vi "main.vi"() -> ()   [LabVIEW 2013]
panel:
  in  "?":enum32{"Movement", "Temprature", "Acceleration"}(tab)
  in  "?":dbl
  in  "?":dbl
  in  "?":dbl
  in  "?":dbl
  in  "?":dbl
  in  "?":dbl
  in  "?":dbl
  in  "?":dbl
  in  "?":dbl
  in  "?":dbl
  in  "?":dbl
  in  "?":dbl
  in  "?":dbl
  in  "?":dbl
  in  "?":dbl
  in  "?":dbl
  out "Ch8 2":dbl
  out "Ch7 2":dbl
  out "Ch6 2":dbl
  out "Ch5 2":dbl
  out "Ch4 2":dbl
  out "Ch3 2":dbl
  out "Ch2 2":dbl
  out "Ch1 2":dbl
  out "?":bool
  in  "?":bool
  in  "?":dbl
  in  "?":dbl
  in  "?":dbl
  in  "?":dbl
  in  "?":dbl
  in  "?":dbl
  in  "?":dbl
  in  "?":dbl
  in  "?":dbl
  in  "?":dbl
  in  "?":dbl
  in  "?":dbl
  in  "?":dbl
  in  "?":dbl
  in  "?":dbl
  in  "?":dbl
  out "Ch8":dbl
  out "Ch7":dbl
  out "Ch6":dbl
  out "Ch5":dbl
  out "Ch4":dbl
  out "Ch3":dbl
  out "Ch2":dbl
  out "Ch1":dbl
  out "Strain Graph":waveform(dbl)(graph)
  out "Live Preview":u8[][](graph)
  in  "Blank Button 6":bool
  in  "?":T1(tab)
  in  "Blank Button 2":bool
  in  "Blank Button":bool
  out "Current Position X & Y (units)":dbl[](array[numeric]) format="%_10e"
  out "Postion After Movment  X & Y (units)":dbl[](array[numeric]) format="%_10e"
  in  "Target Displacement X & Y (units)":dbl[](array[numeric]) format="%_6f"
  in  "?":bool
  in  "?":bool
  out "Best Focus":cluster{"X":dbl, "Y":dbl}[](graph)
  in  "Blank Button 5":bool
  in  "Blank Button 4":bool
  in  "Blank Button 3":bool
  in  "?":bool
  in  "?":bool
  out "Postion After Movment Z":dbl format="%_10e"
  in  "Target Displacement Z":dbl format="%_6f"
  out "Current Position Z":dbl format="%_10e"
  out "String":string
  in  "OK Button 17":bool
  in  "OK Button 16":bool
  in  "Sensors 2":T2(radio)
  in  "OK Button 15":bool
  out "?":dbl[](array[numeric]) format="%.6f"
  in  "OK Button 14":bool
  in  "OK Button 13":bool
  in  "OK Button 12":bool
  in  "OK Button 11":bool
  in  "OK Button 10":bool
  in  "OK Button 9":bool
  in  "OK Button 8":bool
  in  "OK Button 7":bool
  in  "OK Button 6":bool
  in  "OK Button 5":bool
  in  "OK Button 4":bool
  in  "OK Button 3":bool
  in  "OK Button 2":bool
  in  "OK Button":bool
  in  "target w 2":dbl=0.2 format="%.6f"
  in  "target v 2":dbl=0.2 format="%.6f"
  in  "target u 2":dbl=0.2 format="%.6f"
  in  "target z 2":dbl=0.2 format="%.6f"
  in  "target y 2":dbl=0.2 format="%.6f"
  in  "target x 2":dbl=0.2 format="%.6f"
  out "current position 3":dbl[](array[numeric]) format="%.6f"
  out "current position 2":dbl[](array[numeric]) format="%.6f"
  out "current position":dbl[](array[numeric]) format="%.6f"
  out "?":dbl[](array[numeric]) format="%.6f"
  in  "target w":dbl=0.2 format="%.6f"
  in  "target v":dbl=0.2 format="%.6f"
  in  "target u":dbl=0.2 format="%.6f"
  in  "target z":dbl=0.2 format="%.6f"
  in  "target y":dbl=0.2 format="%.6f"
  in  "target x":dbl=0.2 format="%.6f"
  in  "Range w":dbl=0.2 format="%.6f"
  in  "Range v":dbl=0.2 format="%.6f"
  in  "Range u":dbl=0.2 format="%.6f"
  in  "Range z":dbl=0.2 format="%.6f"
  in  "Range y":dbl=0.2 format="%.6f"
  in  "Range x":dbl=0.2 format="%.6f"
  out "Temp Out of Range":bool
  in  "Min Temp":dbl=15.0
  in  "Max Temp":dbl=30.0
  out "Ch32":dbl
  out "Ch31":dbl
  out "Ch30":dbl
  out "Ch29":dbl
  out "Ch28":dbl
  out "Ch27":dbl
  out "Ch26":dbl
  out "Ch25":dbl
  out "Ch24":dbl
  out "Ch23":dbl
  out "Ch22":dbl
  out "Ch21":dbl
  out "Ch20":dbl
  out "Ch19":dbl
  out "Ch18":dbl
  out "Ch17":dbl
  out "Waveform Chart":waveform(dbl)(graph)
  in  "stop":bool
  out "Ch16":dbl
  out "Ch15":dbl
  out "Ch14":dbl
  out "Ch13":dbl
  out "Ch12":dbl
  out "Ch11":dbl
  out "Ch10":dbl
  out "Ch9":dbl
  out "Ch8":dbl
  out "Ch7":dbl
  out "Ch6":dbl
  out "Ch5":dbl
  out "Ch4":dbl
  out "Ch3":dbl
  out "Ch2":dbl
  out "Ch1":dbl
  # "Strain Values"
  # "Channels"
  # "Threshold/max"
  # "Threshold/min"
  # "Reference Position"
  # "Range Axis"
  # "Target Position"
  # "Pre- Position"
  # "Current Position"
  # "Step size"
  # "X axis"
  # "Y axis"
  # "Z axis"
  # "U axis"
  # "V axis"
  # "W axis"
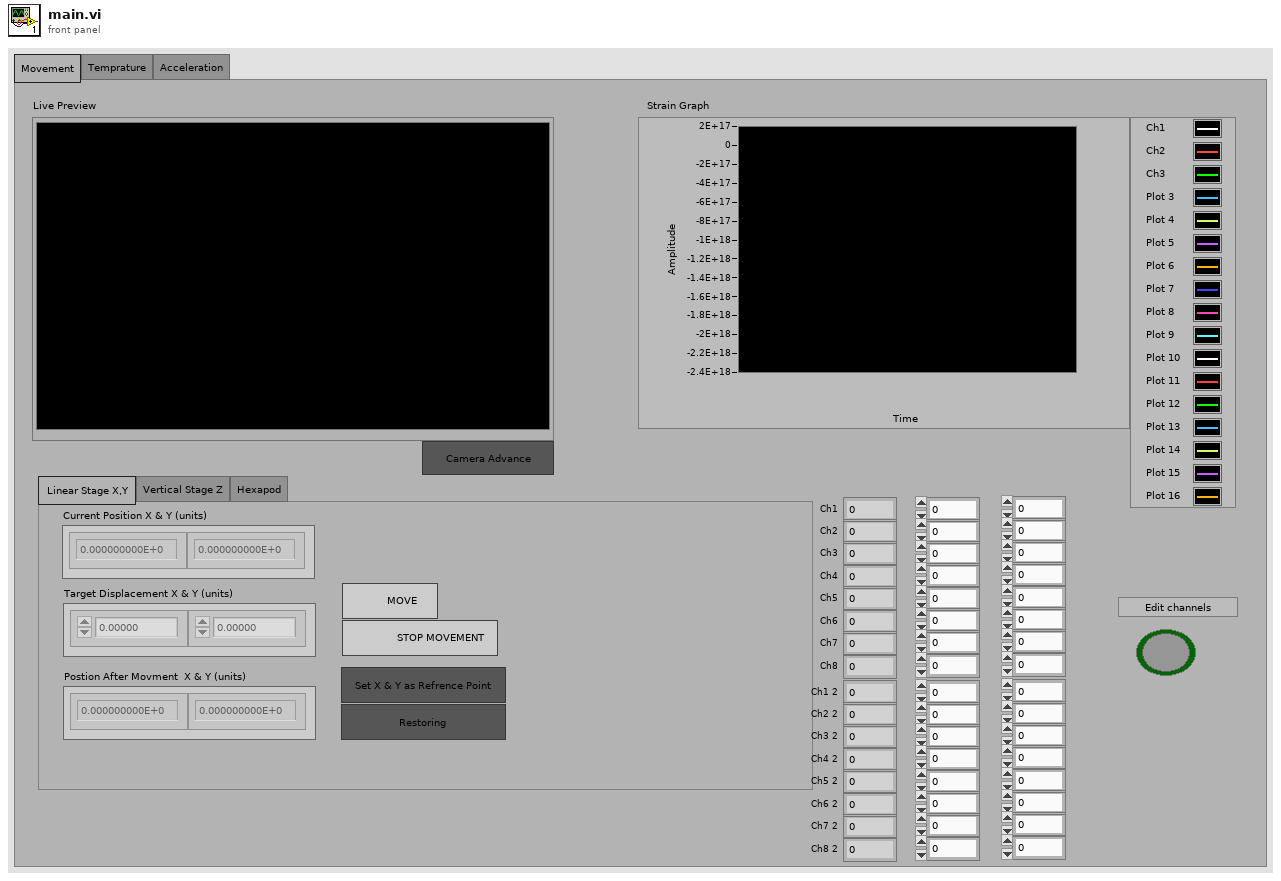
[diagram p1: front panel]
types:
  T1 = enum32{"Linear Stage X,Y ", "Vertical Stage Z", "Hexapod"}
  T2 = enum32{"Radio Selection 2", "Radio Selection 3", "Radio Selection 4", "Radio Selection 5", "Radio Selection 6", "Radio Selection 7"}
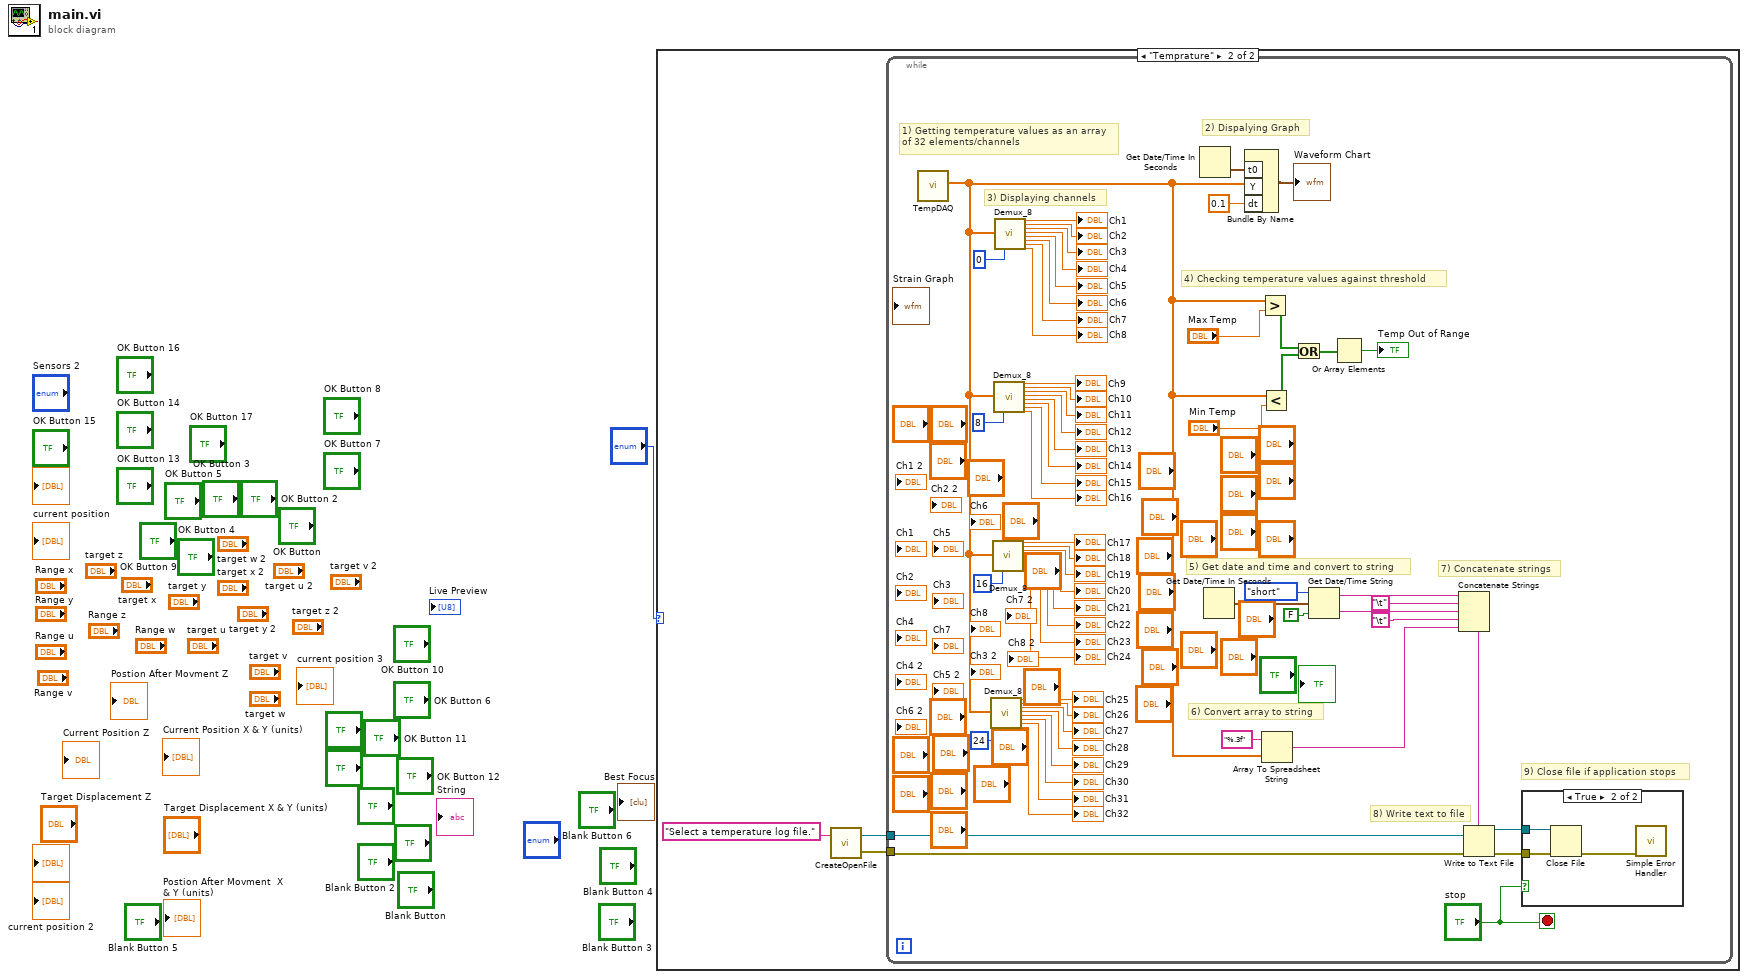
[diagram p0: block diagram]
diagram:
  n1 = case shown="\"Temprature\"" "?" {
    frame "Movement", Default {
    }
    frame "Temprature" {
      n2 = call "CreateOpenFile.vi"("Prompt String"="Select a temperature log file.") -> ("error out"=w2:errorcluster, "refnum out"=w3:refnum<file>)  [unwired: 1 in]
      n3 = while {
        tunnel: w3 -> [w9]
        tunnel: w2 -> [w8]
        stop <- "stop" stop-if-true
        # "8) Write text to file"
        # "9) Close file if application stops"
        # "7) Concatenate strings"
        # "6) Convert array to string"
        # "5) Get date and time and convert to string"
        # "4) Checking temperature values against threshold"
        # "1) Getting temperature values as an array\nof 32 elements/channels"
        # "3) Displaying channels"
        # "2) Dispalying Graph"
        n4 = call "TempDAQ.vi"() -> ("Array"=w20:dbl[])  [unwired: 11 in]
        n5 = call "Demux_8.vi"("Data_Array"=w20, "Index"=24) -> ("element_1"=→"Ch25":dbl, "element_2"=→"Ch26":dbl, "element_3"=→"Ch27":dbl, "element_4"=→"Ch28":dbl, "element_5"=→"Ch29":dbl, "element_6"=→"Ch30":dbl, "element_7"=→"Ch31":dbl, "element_8"=→"Ch32":dbl)  [unwired: 18 in]
        n6 = call "Demux_8.vi"("Data_Array"=w20, "Index"=16) -> ("element_1"=→"Ch17":dbl, "element_2"=→"Ch18":dbl, "element_3"=→"Ch19":dbl, "element_4"=→"Ch20":dbl, "element_5"=→"Ch21":dbl, "element_6"=→"Ch22":dbl, "element_7"=→"Ch23":dbl, "element_8"=→"Ch24":dbl)  [unwired: 18 in]
        n7 = call "Demux_8.vi"("Data_Array"=w20, "Index"=8) -> ("element_1"=→"Ch9":dbl, "element_2"=→"Ch10":dbl, "element_3"=→"Ch11":dbl, "element_4"=→"Ch12":dbl, "element_5"=→"Ch13":dbl, "element_6"=→"Ch14":dbl, "element_7"=→"Ch15":dbl, "element_8"=→"Ch16":dbl)  [unwired: 18 in]
        n8 = call "Demux_8.vi"("Data_Array"=w20, "Index"=0) -> ("element_1"=→"Ch1":dbl, "element_2"=→"Ch2":dbl, "element_3"=→"Ch3":dbl, "element_4"=→"Ch4":dbl, "element_5"=→"Ch5":dbl, "element_6"=→"Ch6":dbl, "element_7"=→"Ch7":dbl, "element_8"=→"Ch8":dbl)  [unwired: 18 in]
        n9 = Get Date/Time In Seconds() -> (seconds since 1Jan1904=w49:timestamp)
        n10 = Get Date/Time In Seconds() -> (seconds since 1Jan1904=w18:timestamp)
        n11 = Bundle By Name("t0"=w49, "Y"=w20, "dt"=0.1) -> (→"Waveform Chart":waveform(dbl))  [unwired: 1 in]
        n12 = Greater?(x=w20, y="Max Temp") -> (0:w24:bool[])
        n13 = Less?(x=w20, y="Min Temp") -> (x < y?=w23:bool[])
        n14 = Array To Spreadsheet String(array=w20, 3:"%.3f" ("format string")) -> (spreadsheet string=w11:string)  [unwired: 1 in]
        n15 = Or(x=w24, y=w23) -> (x .or. y?=w22:bool[])
        n16 = Get Date/Time String(date format (0)=enum16{"short", "long", "abbreviated"}."short", seconds (now)=w18, want seconds? (F)=FALSE) -> (date string=w15:string, time string=w13:string)
        n17 = Or Array Elements(Boolean array=w22) -> (logical OR=→"Temp Out of Range":bool)
        n18 = Concatenate Strings(w15, "\t", w13, "\t", w11) -> (w10:string)
        n19 = Write to Text File(file (use dialog)=w9, text=w10, error in=w8) -> (refnum out=w7:refnum<file>, error out=w6:errorcluster)  [unwired: 1 in, 1 out]
        n20 = case shown="True" "stop" {
          tunnel: w7 -> [_ w68]
          tunnel: w6 -> [_ w67]
          frame False {
          }
          frame True {
            n21 = Close File(refnum=w68, error in=w67) -> (error out=w66:errorcluster)  [unwired: 1 out]
            n22 = call <vilib>:"Simple Error Handler.vi"("error in (no error)"=w66) -> ()  [unwired: 4 in, 5 out]
          }
        }
      }
    }
  }
